vi "_ListAllMDPtrQinMap.vi"(8 "error in":errorcluster, 11 "Variant in":variant) -> (0 "error out":errorcluster, 1 "Array":T1[](array[typedef]), 3 "Variant":variant)   [LabVIEW 2017, in "MDPtr.lvlib" / "MDPtrMgr.lvclass"]
uses:
  MDPtrMgr.lvclass
  Factory/Def-MDPtrQ.ctl
  MDPtr TypeDef/MDPtr DataFrame-Memory.ctl
  MDPtr TypeDef/MDPtr DataFrame-Common.ctl
  <vilib>/Utility/Data Type/Type Definitions/Data Type.ctl
  <vilib>/Utility/Data Type/NI_Data Type.lvlib
  MDPtr.lvlib
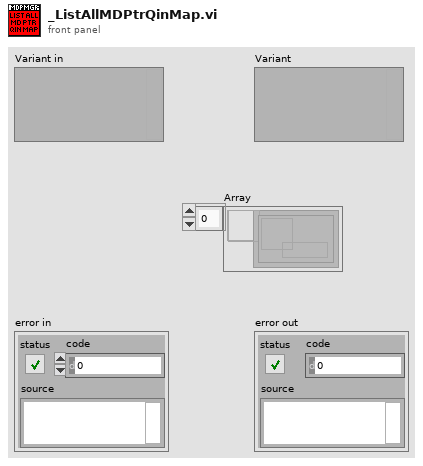
[diagram p1: front panel]
types:
  T1 = typedef "MDPtr.lvlib/MDPtrMgr.lvclass/Def-MDPtrQ.ctl" = refnum<queue>
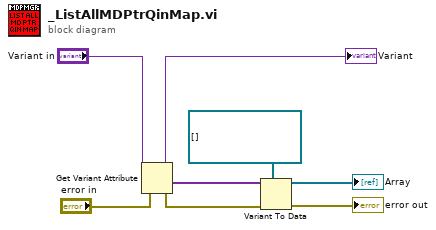
[diagram p0: block diagram]
diagram:
  n1 = Get Variant Attribute(Variant="Variant in", error in="error in") -> (duplicate Variant=→"Variant":variant, values=w5:variant[], error out=w1:errorcluster)  [unwired: 2 in, 1 out]
  n2 = Variant To Data(error in=w1, type=T1[] [] ("Array"), Variant=w5) -> (data=→"Array":T1[], error out=→"error out":errorcluster)
